vi "Get SLSC Module Resource.vi"(8 "error in (no error)":errorcluster, 11 "SLSC Module":T1 format="%.0x") -> (0 "error out":errorcluster, 2 "SLSC Module Resource":refnum<k21>, 3 "SLSC Module out":T1 format="%.0x")   [LabVIEW 2020, in "VeriStand SLSC Scripting.lvlib"]
uses:
  VeriStand SLSC Scripting.lvlib
  <vilib>/NI VeriStand/Custom Device API/Custom Device Item Ref.ctl
  <vilib>/NI VeriStand/Custom Device API/Get Item Property (I32).vi
  <vilib>/NI VeriStand/Custom Device API/Custom Device API.lvlib
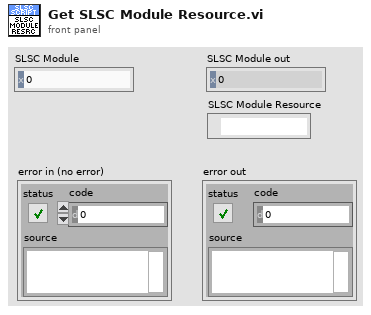
[diagram p1: front panel]
types:
  T1 = typedef "Custom Device API.lvlib/Custom Device Item Ref.ctl" = u64
  T2 = typedef "VeriStand SLSC Scripting.lvlib/SLSC Chassis ID.ctl" = cluster{"Name or IP":string, "ChassisIDType":i32, "chassisType":i32}
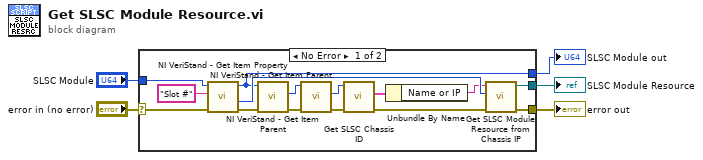
[diagram p0: block diagram]
diagram:
  n1 = case shown="No Error" "error in (no error)" {
    selector: "error in (no error)" -> [w19 w22]
    tunnel: [w17 _] -> w4
    tunnel: "SLSC Module" -> [w16 w21]
    tunnel: [w15 w22] -> w2
    tunnel: [w10 w21] -> w1
    frame No Error {
      n2 = call-poly <vilib>:"NI VeriStand - Get Item Property.vi"("error in (no error)"=w19, "Property Name"="Slot #", "Item Ref in"=w16) -> ("error out"=w11:errorcluster, "Value"=w18:i32, "Item Ref out"=w10:T1)  [unwired: 5 in, 1 out]
      n3 = call <vilib>:"NI VeriStand - Get Item Parent.vi"("error in (no error)"=w11, "Item Ref in"=w10) -> ("error out"=w12:errorcluster, "Parent Ref"=w9:T1)  [unwired: 6 in, 2 out]
      n4 = call <vilib>:"NI VeriStand - Get Item Parent.vi"("error in (no error)"=w12, "Item Ref in"=w9) -> ("error out"=w13:errorcluster, "Parent Ref"=w8:T1)  [unwired: 6 in, 2 out]
      n5 = call "Get SLSC Chassis ID.vi"("error in (no error)"=w13, "SLSC Chassis Ref in"=w8) -> ("error out"=w14:errorcluster, "SLSC Chassis ID"=w7:T2)  [unwired: 7 in, 1 out]
      n6 = Unbundle By Name(w7) -> ("Name or IP"=w6:string)
      n7 = call "Get SLSC Module Resource from Chassis IP.vi"("error in (no error)"=w14, "Slot Number"=w18, "Chassis Name or IP"=w6) -> ("error out"=w15:errorcluster, "SLSC Device"=w17:refnum<k21>)  [unwired: 7 in]
    }
    frame Error {
    }
  }
  "SLSC Module Resource" <- w4
  "SLSC Module out" <- w1
  "error out" <- w2
